vi "CLD 6 CSV file utility.vi"(8 "Fehler (Eingang)":T1, 10 "[Daten, Eingang]":T2[](array[typedef])=[{"Verweildauer"=3, "Zustand 1"=TRUE, "Zustand 2"=FALSE, "Zustand 3"=FALSE}, {"Verweildauer"=4, "Zustand 1"=FALSE, "Zustand 2"=TRUE, "Zustand 3"=FALSE}, {"Verweildauer"=5, "Zustand 1"=FALSE, "Zustand 2"=FALSE, "Zustand 3"=TRUE}], 11 "CSV lesen/CSV schreiben":T3) -> (0 "Fehler (Ausgang)":T1, 3 "[Daten, Ausgang]":T2[](array[typedef]))   [LabVIEW 2014]
doc: "CLD-Übung 6"
uses:
  CLD 6 CSV file enum.ctl
  CLD 6 CSV file data structure.ctl
panel:
  out "Hinzugefügter Pfad":path
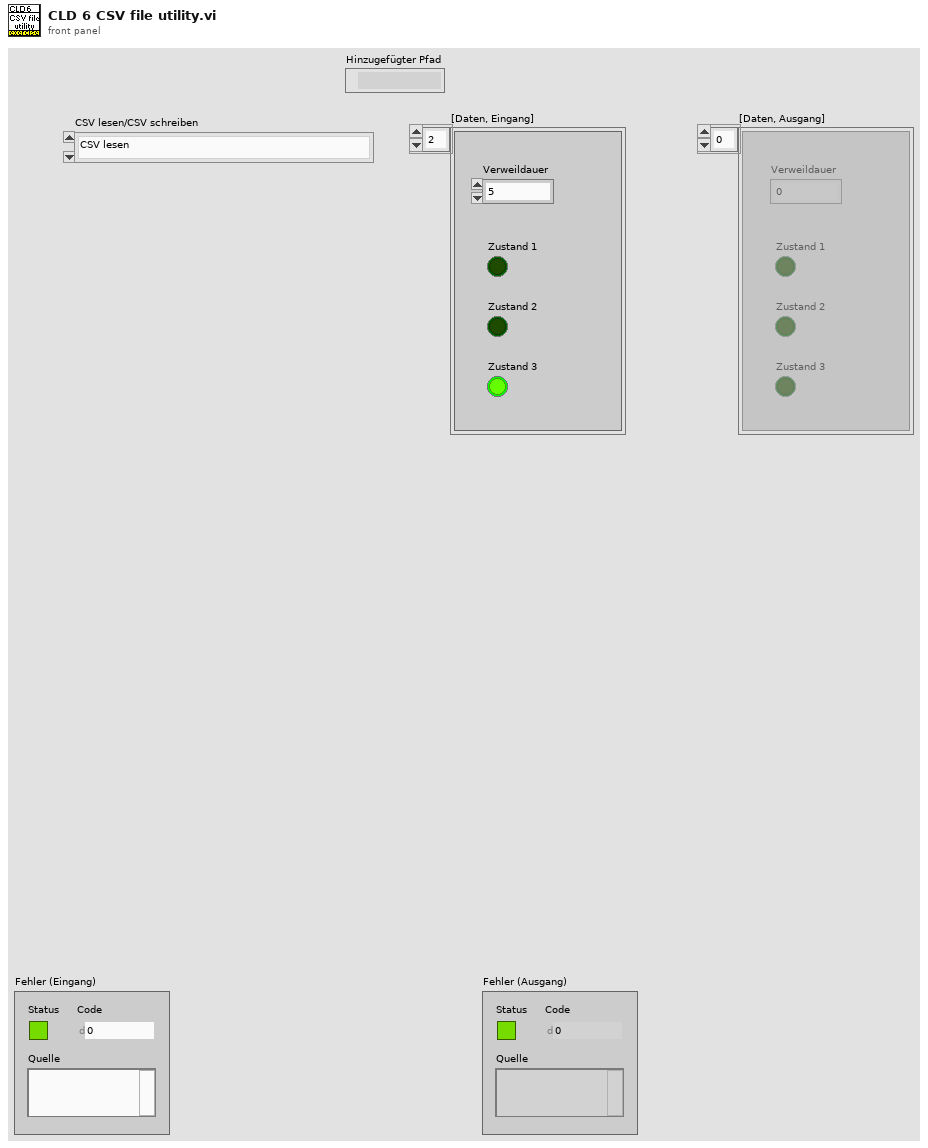
[diagram p1: front panel]
types:
  T1 = cluster{"Status":bool, "Code":i32, "Quelle":string}
  T2 = typedef "CLD 6 CSV file data structure.ctl" = cluster{"Verweildauer":i32, "Zustand 1":bool, "Zustand 2":bool, "Zustand 3":bool}
  T3 = typedef "CLD 6 CSV file enum.ctl" = enum16{"CSV lesen", "CSV schreiben"}
  T4 = enum16{"open", "replace", "create", "open or create", "replace or create", "replace or create with confirmation"}
  T5 = cluster{"[0]":bool, "[1]":bool, "[2]":bool, "[3]":bool, "[4]":bool, "[5]":bool, "[6]":bool, "[7]":bool, "[8]":bool}
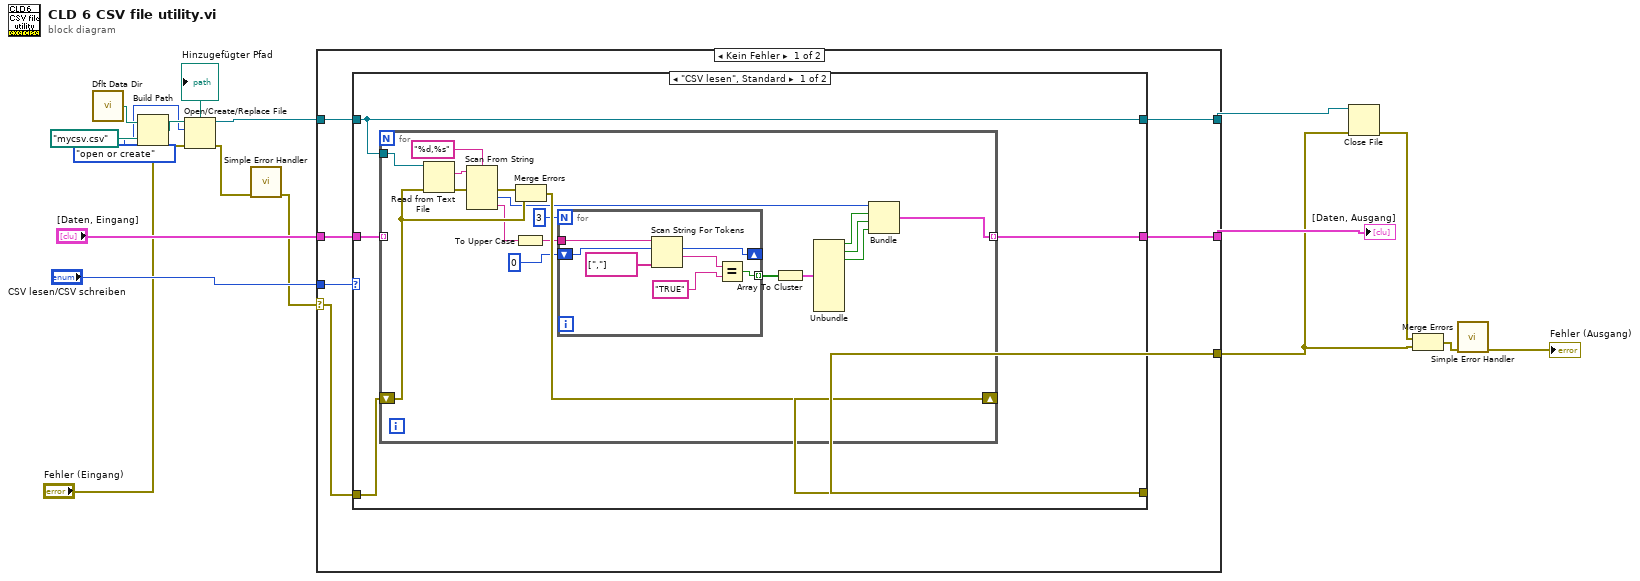
[diagram p0: block diagram]
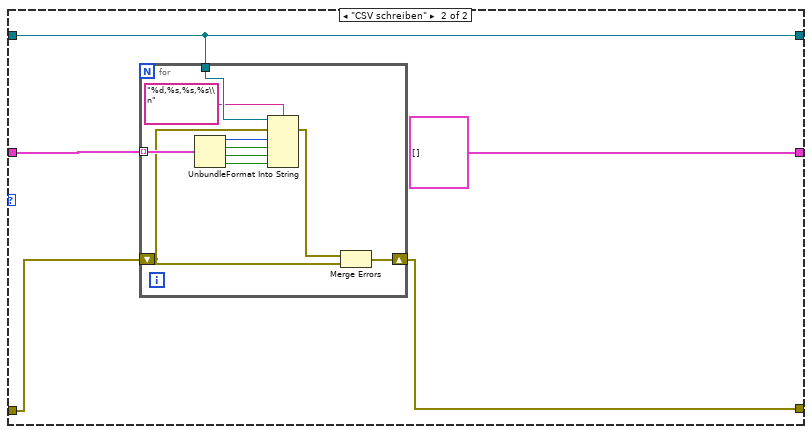
[diagram p2: hidden frame]
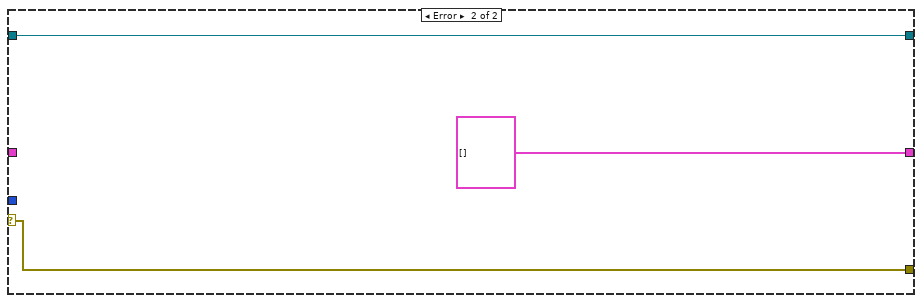
[diagram p3: hidden frame]
diagram:
  n1 = call <vilib>:"Dflt Data Dir.vi"() -> ("App:Default Data Directory"=w14:path)
  n2 = Build Path(base path=w14, name or relative path=path "mycsv.csv" ("default name")) -> (appended path=w8:path)
  "Hinzugefügter Pfad" <- w8
  n3 = Open/Create/Replace File(file path (use dialog)=w8, error in="Fehler (Eingang)", operation (0:open)=T4."open or create" ("Operation (0:Öffnen)")) -> (refnum out=w9:refnum<file>, error out=w10:errorcluster)  [unwired: 3 in, 1 out]
  n4 = call <vilib>:"Simple Error Handler.vi"("error in (no error)"=w10) -> ("error out"=w4:errorcluster)  [unwired: 4 in, 4 out]
  n5 = case shown="Kein Fehler" w4 {
    selector: w4 -> [w17 w71]
    tunnel: "CSV lesen/CSV schreiben" -> [w23 _]
    tunnel: "[Daten, Eingang]" -> [w22 _]
    tunnel: [w21 w71] -> w1
    tunnel: w9 -> [w20 w69]
    tunnel: [w19 w69] -> w6
    tunnel: [w18 T2[] []] -> w5
    frame No Error {
      n6 = case shown="\"CSV lesen\", Standard" w23 {
        tunnel: w22 -> [w24 w55]
        tunnel: w17 -> [w27 w56]
        tunnel: w20 -> [w25 w58]
        tunnel: [w25 w58] -> w19
        tunnel: [w26 w57] -> w21
        tunnel: [w28 T2[] []] -> w18
        frame "CSV lesen", Default {
          n7 = for {
            tunnel: w25 -> [w44]
            tunnel: [w46] -> w28 mode=indexing
            shift-right: [w45] -> w26
            shift-left: w27 -> [w43]
            tunnel: w24 -> [_] mode=indexing
            n8 = Read from Text File(file (use dialog)=w44, error in=w43) -> (text=w38:string, error out=w41:errorcluster)  [unwired: 2 in, 2 out]
            n9 = Scan From String(format string="%d,%s" ("Format-String"), input string=w38, error in=w41) -> (error out=w39:errorcluster, output 1=w40:i32, output 2=w32:string)  [unwired: 3 in, 2 out]
            n10 = To Upper Case(1:w32) -> (0:w31:string)
            n11 = Merge Errors(w39, w43) -> (w45:errorcluster)
            n12 = for {
              N: 3 -> [_]
              tunnel: w31 -> [w50]
              shift-right: [w51] -> _
              shift-left: 0 ("offset past token") -> [w52]
              tunnel: [w47] -> w29 mode=indexing
              n13 = Scan String For Tokens(6:string[] [","] ("Trennzeichen (\\s,\\t,\\r,\\n)"), 8:w52, 9:w50) -> (1:w49:string, 2:w51:i32)  [unwired: 3 in, 2 out]
              n14 = Equal?(x=w49, y="TRUE" ("True-String")) -> (x = y?=w47:bool)
            }
            n15 = Array To Cluster(array=w29) -> (cluster=w37:T5)
            n16 = Unbundle(w37) -> ("[0]"=w36:bool, "[1]"=w35:bool, "[2]"=w34:bool)  [unwired: 6 out]
            n17 = Bundle(w40, "[0]"=w36, "[1]"=w35, "[2]"=w34) -> (w46:cluster{i32, "[0]":bool, "[1]":bool, "[2]":bool})  [unwired: 1 in]
          }
        }
        frame "CSV schreiben" {
          n18 = for {
            tunnel: w55 -> [w68] mode=indexing
            tunnel: w58 -> [w66]
            shift-right: [w67] -> w57
            shift-left: w56 -> [w65]
            n19 = Unbundle(w68) -> ("Verweildauer"=w63:i32, "Zustand 1"=w62:bool, "Zustand 2"=w61:bool, "Zustand 3"=w60:bool)
            n20 = Format Into String(format string="%d,%s,%s,%s\\n" ("Format-String"), initial string=w66, error in=w65, w63, w62, w61, w60) -> (error out=w59:errorcluster)  [unwired: 1 out]
            n21 = Merge Errors(w59, w65) -> (w67:errorcluster)
          }
        }
      }
    }
    frame Error {
    }
  }
  "[Daten, Ausgang]" <- w5
  n22 = Close File(refnum=w6, error in=w1) -> (error out=w2:errorcluster)  [unwired: 1 out]
  n23 = Merge Errors(w2, w1) -> (w3:errorcluster)
  n24 = call <vilib>:"Simple Error Handler.vi"("error in (no error)"=w3) -> ("error out"=→"Fehler (Ausgang)":errorcluster)  [unwired: 4 in, 4 out]
